vi "loop_transistor.vi"() -> ()   [LabVIEW 2020]
uses:
  <vilib>/Analysis/baseanly.llb/Mean (DBL).vi
  <vilib>/Utility/file.llb/Write Delimited Spreadsheet (DBL).vi
  <vilib>/Analysis/NI_AALBase.lvlib
panel:
  out "Isc [mA]":dbl
  out "Voc [V]":dbl
  out "resistance_MPP [kohm]":dbl
  out "resistance [kohm]":dbl
  in  "Save MPP operation data?":bool=TRUE
  out "MPP operating data log path":string
  in  "MPP operating\nfile name":string="MPP_operating"
  out "MPP tracking data log path":string
  in  "Save MPP tracking data?":bool=TRUE
  in  "MPP tracking\nfile name":string="MPP_tracking"
  in  "# points \nMPP operation":i32=6
  out "# iterations \nMPP operation (2nd loop)":dbl
  out "# iterations \nMPP tracking (1st loop)":i32
  out "error out":errorcluster
  out "Vgs_MPP [V]":dbl
  out "V_MPP [V]":dbl
  out "I_MPP [mA]":dbl
  out "index max power":i32
  out "max power [mW]":dbl
  in  "STOP":bool
  out "power [mW]":dbl
  in  "Tab Control":T1(tab)
  out "IV-PV":cluster{dbl[], dbl[]}[](graph)
  out "Power":dbl[](graph)
  out "Resistance-Vgs":cluster{dbl[], dbl[]}(graph)
  out "I,V (Vgs)":cluster{dbl[], dbl[]}[](graph)
  out "IV-PV":cluster{dbl[], dbl[]}[](graph)
  out "Current-Voltage-Power operating":dbl[][](graph)
  out "voltage [V]":dbl format="%0.2f"
  out "current [mA]":dbl
  in  "# points\nMPP tracking":i32=3
  out "Vgs [V]":dbl
  in  "Vgs stop":dbl=4.0 format="%#_13g"
  in  "Vgs step":dbl=0.05 format="%#_13g"
  in  "Vgs start":dbl=3.0 format="%#_13g"
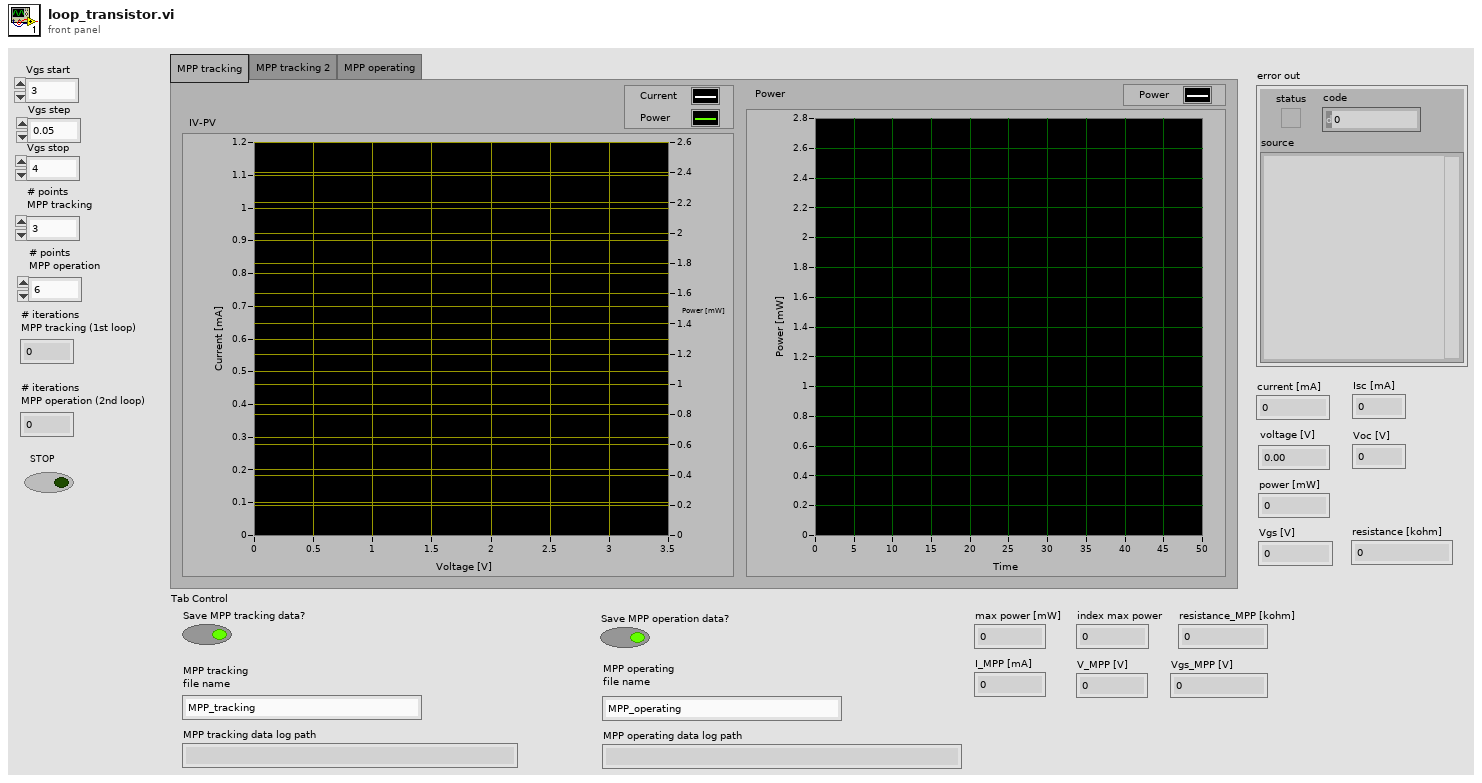
[diagram p1: front panel]
types:
  T1 = enum32{"MPP tracking", "MPP tracking 2", "MPP operating"}
  T2 = enum16{"open", "replace", "create", "open or create", "replace or create", "replace or create with confirmation"}
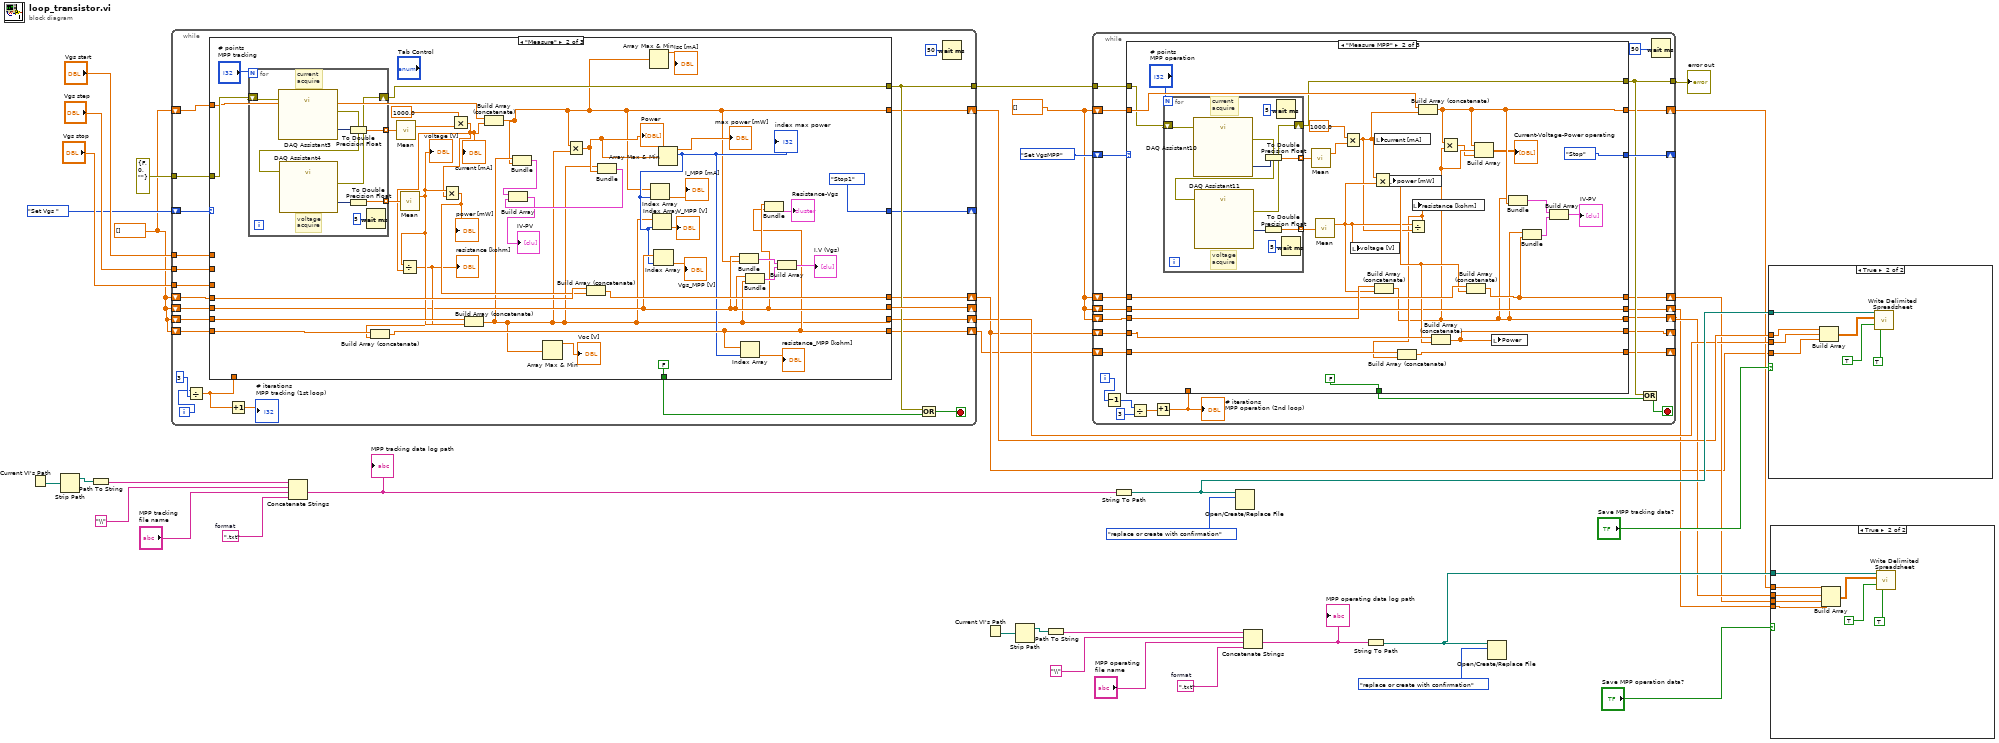
[diagram p0: block diagram]
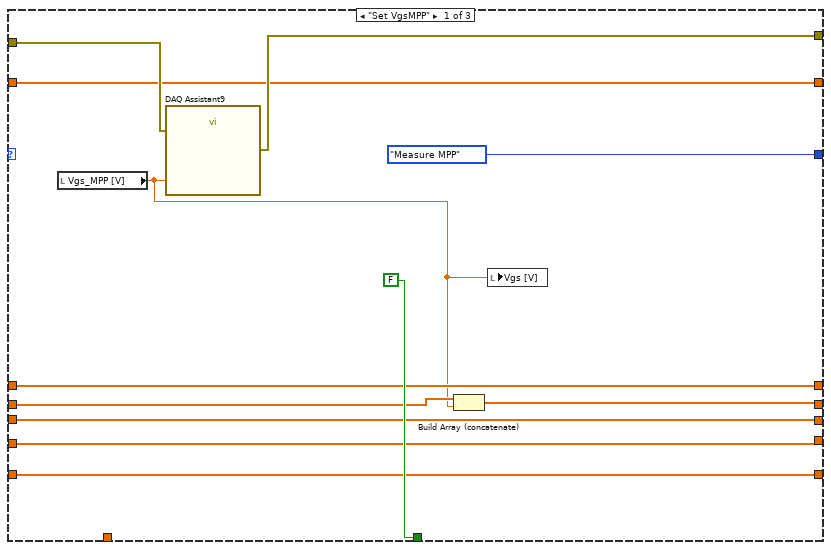
[diagram p4: hidden frame]
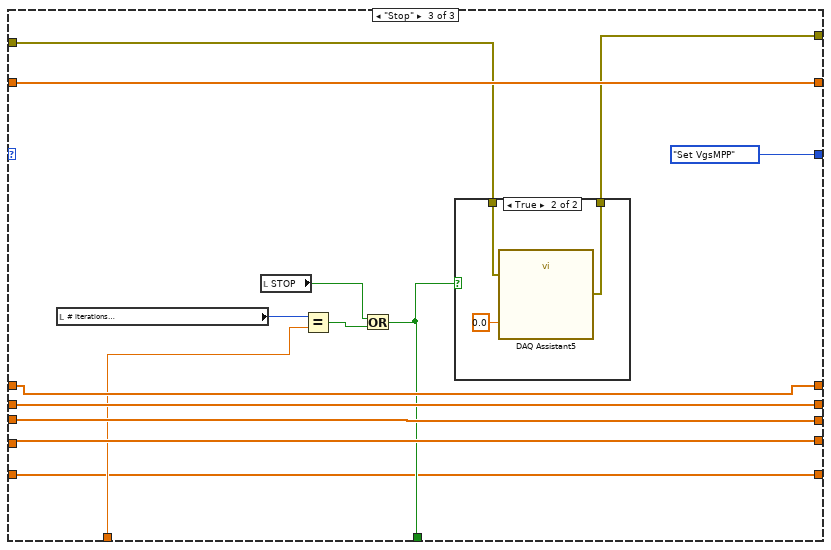
[diagram p5: hidden frame]
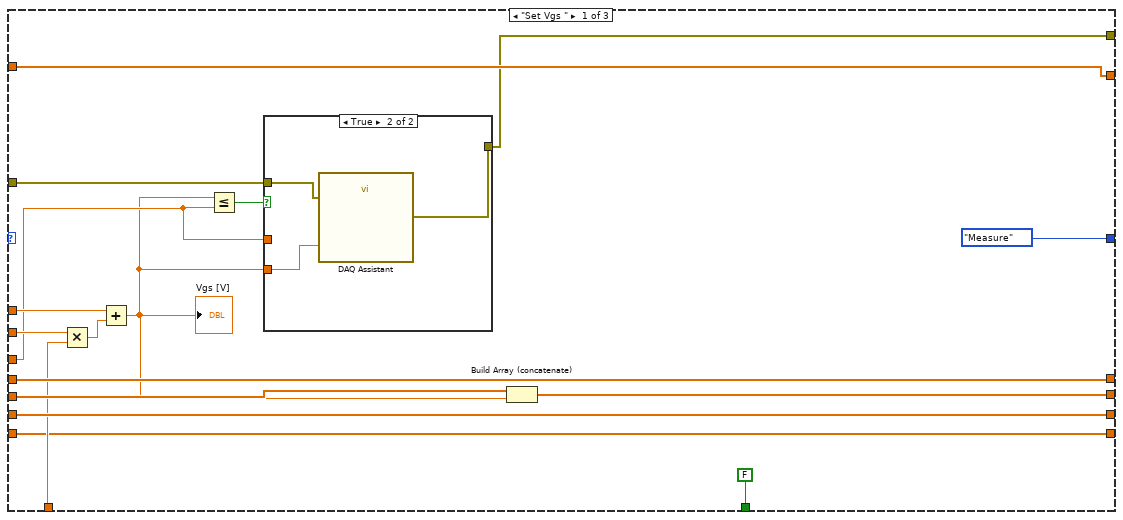
[diagram p7: hidden frame]
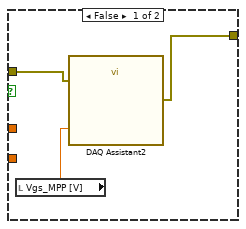
[diagram p8: hidden frame]
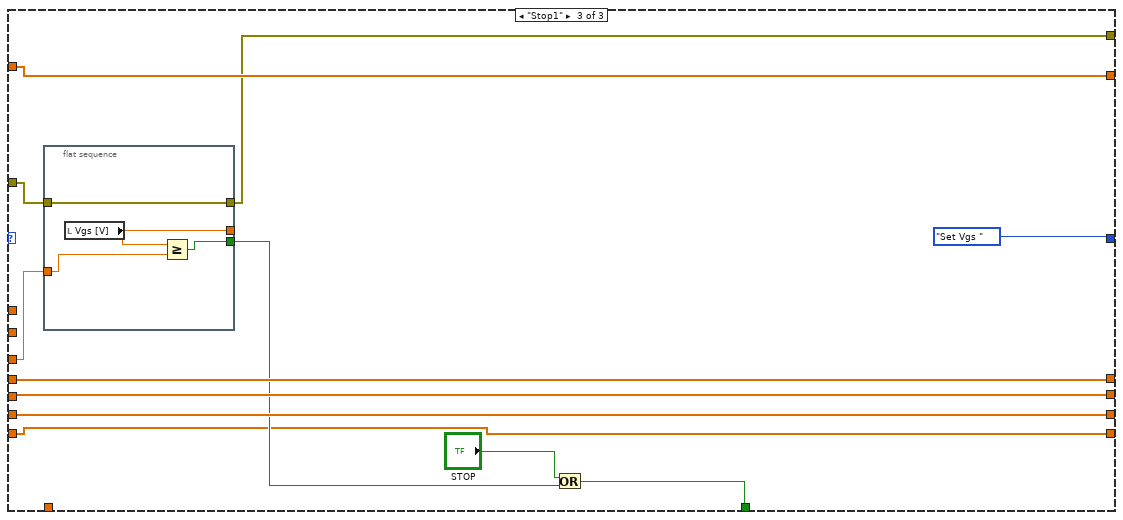
[diagram p9: hidden frame]
diagram:
  w14 = ".txt"  # format
  w26 = ".txt"  # format
  w32 = dbl[] []
  w2 = dbl[] []
  n1 = Current VI's Path() -> (path=w18:path)
  n2 = Strip Path(path=w18) -> (stripped path=w19:path)  [unwired: 1 out]
  n3 = Path To String(path=w19) -> (string=w29:string)
  n4 = while {
    tunnel: "Vgs start" -> [w62]
    tunnel: "Vgs step" -> [w61]
    tunnel: "Vgs stop" -> [w60]
    tunnel: errorcluster {"status"=FALSE, "code"=0, "source"=""} ("error in") -> [w59]
    tunnel: [w55] -> w31
    shift-right: [w57] -> _
    shift-left: w2 -> [w58]
    shift-right: [w45] -> _
    shift-left: enum16{"Set Vgs ", "Measure", "Stop1"}."Set Vgs " -> [w52]
    shift-right: [w50] -> w21
    shift-left: w2 -> [w51]
    shift-right: [w48] -> w20
    shift-left: w2 -> [w49]
    shift-right: [w46] -> w3
    shift-left: w2 -> [w47]
    shift-right: [w39] -> w1
    shift-left: w2 -> [w40]
    i -> [w43]
    stop <- w56 stop-if-true
    n5 = Divide(x=w43, y=3) -> (x/y=w41:dbl)
    n6 = case shown="\"Measure\"" w52 {
      tunnel: [enum16{"Set Vgs ", "Measure", "Stop1"}."Measure" enum16{"Set Vgs ", "Measure", "Stop1"}."Stop1" enum16{"Set Vgs ", "Measure", "Stop1"}."Set Vgs "] -> w45
      tunnel: w62 -> [w77 _ _]
      tunnel: w61 -> [w79 _ _]
      tunnel: w60 -> [w67 _ w141]
      tunnel: w41 -> [w66 _ _]
      tunnel: w59 -> [w75 w121 w140]
      tunnel: [w64 w122 w133] -> w55
      tunnel: w58 -> [w74 w94 w138]
      tunnel: [w73 w94 w138] -> w57
      tunnel: [FALSE FALSE w134] -> w54
      tunnel: w51 -> [w70 w116 w143]
      tunnel: [w70 w87 w143] -> w50
      tunnel: w49 -> [w71 w115 w137]
      tunnel: [w71 w89 w137] -> w48
      tunnel: w47 -> [w69 w110 w139]
      tunnel: [w69 w108 w139] -> w46
      tunnel: w40 -> [w63 w96 w132]
      tunnel: [w63 w92 w132] -> w39
      frame "Set Vgs " {
        n7 = Multiply(x=w79, y=w66) -> (x*y=w78:dbl)
        n8 = Add(x=w77, y=w78) -> (x+y=w65:dbl)
        "Vgs [V]" <- w65
        n9 = Less Or Equal?(x=w65, y=w67) -> (x <= y?=w76:bool)
        n10 = case shown="True" w76 {
          tunnel: w65 -> [_ w85]
          tunnel: w75 -> [w82 w84]
          tunnel: w67 -> [_ _]
          tunnel: [w81 w83] -> w64
          frame False {
            n11 = local read "Vgs_MPP [V]"() -> (w80:dbl)
            n12 = call "DAQ Assistant2"("data"=w80, "error in"=w82) -> ("error out"=w81:errorcluster)  [unwired: 16 in, 1 out]
          }
          frame True {
            n13 = call "DAQ Assistant"("data"=w85, "error in"=w84) -> ("error out"=w83:errorcluster)  [unwired: 16 in, 1 out]
          }
        }
        n14 = Build Array (concatenate)(w74, w65) -> (w73:dbl[])
      }
      frame "Measure" {
        n15 = for {
          N: "# points\nMPP tracking" -> [_]
          shift-right: [w130] -> w122
          shift-left: w121 -> [w126]
          tunnel: [w125] -> w120 mode=indexing
          tunnel: [w124] -> w117 mode=indexing
          # "voltage\nacquire"
          # "current \nacquire"
          n16 = call "DAQ Assistant3"("error in"=w126) -> ("data"=w128:dynamicdata, "error out"=w131:errorcluster)  [unwired: 16 in, 1 out]
          n17 = call "DAQ Assistant4"("error in"=w131) -> ("data"=w127:dynamicdata, "error out"=w130:errorcluster)  [unwired: 16 in, 1 out]
          n18 = To Double Precision Float(number=w128) -> (double precision float=w125:dbl)
          n19 = To Double Precision Float(number=w127) -> (double precision float=w124:dbl)
          n20 = Wait (ms)(milliseconds to wait=u32 5) -> ()  [unwired: 1 out]
        }
        n21 = call-poly <vilib>:"Mean.vi"("X"=w120) -> ("mean"=w119:dbl)  [unwired: 1 out]
        n22 = call-poly <vilib>:"Mean.vi"("X"=w117) -> ("mean"=w98:dbl)  [unwired: 1 out]
        "voltage [V]" <- w98
        n23 = Multiply(x=1000.0, y=w119) -> (x*y=w97:dbl)
        "current [mA]" <- w97
        n24 = Divide(x=w98, y=w97) -> (x/y=w95:dbl)
        "resistance [kohm]" <- w95
        n25 = Build Array (concatenate)(w96, w95) -> (w92:dbl[])
        n26 = Multiply(x=w98, y=w97) -> (x*y=w109:dbl)
        "power [mW]" <- w109
        n27 = Build Array (concatenate)(w115, w98) -> (w89:dbl[])
        n28 = Build Array (concatenate)(w116, w97) -> (w87:dbl[])
        n29 = Bundle(w89, w87) -> (w114:cluster{dbl[], dbl[]})  [unwired: 1 in]
        n30 = Array Max & Min(array=w89) -> (max value=→"Voc [V]":dbl)  [unwired: 3 out]
        n31 = Multiply(x=w87, y=w89) -> (x*y=w102:dbl[])
        "Power" <- w102
        n32 = Build Array (concatenate)(w110, w109) -> (w108:dbl[])
        n33 = Bundle(w89, w102) -> (w113:cluster{dbl[], dbl[]})  [unwired: 1 in]
        n34 = Build Array(w114, w113) -> (→"IV-PV":cluster{dbl[], dbl[]}[])
        n35 = Array Max & Min(array=w87) -> (max value=→"Isc [mA]":dbl)  [unwired: 3 out]
        n36 = Array Max & Min(array=w102) -> (max value=→"max power [mW]":dbl, max index (indices)=w91:i32)  [unwired: 2 out]
        "index max power" <- w91
        n37 = Index Array(array=w87, index=w91) -> (element=→"I_MPP [mA]":dbl)
        n38 = Index Array(array=w89, index=w91) -> (element=→"V_MPP [V]":dbl)
        n39 = Index Array(array=w94, index=w91) -> (element=→"Vgs_MPP [V]":dbl)
        n40 = Bundle(w94, w87) -> (w101:cluster{dbl[], dbl[]})  [unwired: 1 in]
        n41 = Index Array(array=w92, index=w91) -> (element=→"resistance_MPP [kohm]":dbl)
        n42 = Bundle(w94, w89) -> (w100:cluster{dbl[], dbl[]})  [unwired: 1 in]
        n43 = Bundle(w94, w92) -> (→"Resistance-Vgs":cluster{dbl[], dbl[]})  [unwired: 1 in]
        n44 = Build Array(w101, w100) -> (→"I,V (Vgs)":cluster{dbl[], dbl[]}[])
      }
      frame "Stop1" {
        n45 = flat-sequence {
          tunnel: w141 -> [w147]
          tunnel: [w146] -> w135
          tunnel: [w145] -> _
          tunnel: w140 -> [w144]
          tunnel: [w144] -> w133
          frame #0 {
            n46 = local read "Vgs [V]"() -> (w145:dbl)
            n47 = Greater Or Equal?(x=w145, y=w147) -> (x >= y?=w146:bool)
          }
        }
        n48 = Or(x="STOP", y=w135) -> (x .or. y?=w134:bool)
      }
    }
    n49 = Increment(x=w41) -> (x+1=→"# iterations \nMPP tracking (1st loop)":dbl)
    n50 = Or(x=w55, y=w54) -> (x .or. y?=w56:bool)
    n51 = Wait (ms)(milliseconds to wait=u32 50) -> ()  [unwired: 1 out]
  }
  n52 = Concatenate Strings(w29, "\\" ("string"), "MPP tracking\nfile name", w26) -> (w25:string)
  "MPP tracking data log path" <- w25
  n53 = Current VI's Path() -> (path=w12:path)
  n54 = Strip Path(path=w12) -> (stripped path=w13:path)  [unwired: 1 out]
  n55 = Path To String(path=w13) -> (string=w17:string)
  n56 = while {
    shift-right: [w170] -> _
    shift-left: enum16{"Set VgsMPP", "Measure MPP", "Stop"}."Set VgsMPP" -> [w171]
    tunnel: [w167] -> w30
    tunnel: w31 -> [w166]
    shift-right: [w164] -> w5
    shift-left: w32 -> [w165]
    shift-right: [w163] -> w6
    shift-left: w32 -> [w162]
    shift-right: [w160] -> w7
    shift-left: w32 -> [w161]
    shift-right: [w158] -> w4
    shift-left: w32 -> [w159]
    shift-right: [w152] -> _
    shift-left: w3 -> [w153]
    shift-right: [w148] -> _
    shift-left: w1 -> [w149]
    i -> [w154]
    stop <- w168 stop-if-true
    n57 = Decrement(x=w154) -> (x-1=w155:i32)
    n58 = Divide(x=w155, y=3) -> (x/y=w156:dbl)
    n59 = Increment(x=w156) -> (x+1=w151:dbl)
    "# iterations \nMPP operation (2nd loop)" <- w151
    n60 = case shown="\"Measure MPP\"" w171 {
      tunnel: [enum16{"Set VgsMPP", "Measure MPP", "Stop"}."Measure MPP" enum16{"Set VgsMPP", "Measure MPP", "Stop"}."Stop" enum16{"Set VgsMPP", "Measure MPP", "Stop"}."Set VgsMPP"] -> w170
      tunnel: [w182 w204 w229] -> w167
      tunnel: [FALSE FALSE w223] -> w150
      tunnel: w166 -> [w180 w202 w230]
      tunnel: [w179 w197 w233] -> w164
      tunnel: w165 -> [w179 w203 w233]
      tunnel: [w178 w186 w232] -> w163
      tunnel: w162 -> [w178 w205 w232]
      tunnel: [w177 w187 w234] -> w160
      tunnel: w161 -> [w177 w206 w234]
      tunnel: w159 -> [w176 w189 w231]
      tunnel: [w175 w189 w231] -> w158
      tunnel: w153 -> [w173 w196 w228]
      tunnel: [w173 w194 w228] -> w152
      tunnel: w151 -> [_ _ w226]
      tunnel: w149 -> [w172 w191 w222]
      tunnel: [w172 w188 w222] -> w148
      frame "Set VgsMPP" {
        n61 = local read "Vgs_MPP [V]"() -> (w174:dbl)
        n62 = call "DAQ Assistant9"("data"=w174, "error in"=w180) -> ("error out"=w182:errorcluster)  [unwired: 16 in, 1 out]
        n63 = Build Array (concatenate)(w176, w174) -> (w175:dbl[])
        n64 = local write "Vgs [V]"(w174) -> ()
      }
      frame "Measure MPP" {
        n65 = for {
          N: "# points \nMPP operation" -> [_]
          shift-right: [w220] -> w204
          shift-left: w202 -> [w216]
          tunnel: [w215] -> w207 mode=indexing
          tunnel: [w214] -> w208 mode=indexing
          # "voltage\nacquire"
          # "current \nacquire"
          n66 = call "DAQ Assistant10"("error in"=w216) -> ("data"=w218:dynamicdata, "error out"=w221:errorcluster)  [unwired: 16 in, 1 out]
          n67 = call "DAQ Assistant11"("error in"=w221) -> ("data"=w217:dynamicdata, "error out"=w220:errorcluster)  [unwired: 16 in, 1 out]
          n68 = To Double Precision Float(number=w218) -> (double precision float=w215:dbl)
          n69 = To Double Precision Float(number=w217) -> (double precision float=w214:dbl)
          n70 = Wait (ms)(milliseconds to wait=u32 5) -> ()  [unwired: 1 out]
          n71 = Wait (ms)(milliseconds to wait=u32 5) -> ()  [unwired: 1 out]
        }
        n72 = call-poly <vilib>:"Mean.vi"("X"=w207) -> ("mean"=w209:dbl)  [unwired: 1 out]
        n73 = call-poly <vilib>:"Mean.vi"("X"=w208) -> ("mean"=w193:dbl)  [unwired: 1 out]
        n74 = Multiply(x=1000.0, y=w209) -> (x*y=w192:dbl)
        n75 = local write "voltage [V]"(w193) -> ()
        n76 = Multiply(x=w192, y=w193) -> (x*y=w195:dbl)
        n77 = local write "current [mA]"(w192) -> ()
        n78 = Build Array (concatenate)(w205, w193) -> (w186:dbl[])
        n79 = local write "power [mW]"(w195) -> ()
        n80 = Divide(x=w193, y=w192) -> (x/y=w190:dbl)
        n81 = Build Array (concatenate)(w191, w190) -> (w188:dbl[])
        n82 = local write "resistance [kohm]"(w190) -> ()
        n83 = Build Array (concatenate)(w206, w192) -> (w187:dbl[])
        n84 = Build Array (concatenate)(w196, w195) -> (w194:dbl[])
        n85 = Multiply(x=w187, y=w186) -> (x*y=w185:dbl[])
        n86 = Build Array (concatenate)(w203, w195) -> (w197:dbl[])
        n87 = Build Array(w187, w186, w185) -> (→"Current-Voltage-Power operating":dbl[][])
        n88 = local write "Power"(w194) -> ()
        n89 = Bundle(w186, w187) -> (w200:cluster{dbl[], dbl[]})  [unwired: 1 in]
        n90 = Bundle(w186, w197) -> (w199:cluster{dbl[], dbl[]})  [unwired: 1 in]
        n91 = Build Array(w200, w199) -> (→"IV-PV":cluster{dbl[], dbl[]}[])
      }
      frame "Stop" {
        n92 = local read "# iterations \nMPP tracking (1st loop)"() -> (w227:i32)
        n93 = local read "STOP"() -> (w225:bool)
        n94 = Equal?(x=w227, y=w226) -> (x = y?=w224:bool)
        n95 = Or(x=w225, y=w224) -> (x .or. y?=w223:bool)
        n96 = case shown="True" w223 {
          tunnel: w230 -> [w236 w239]
          tunnel: [w236 w238] -> w229
          frame False {
          }
          frame True {
            n97 = call "DAQ Assistant5"("data"=0.0, "error in"=w239) -> ("error out"=w238:errorcluster)  [unwired: 16 in, 1 out]
          }
        }
      }
    }
    n98 = Or(x=w167, y=w150) -> (x .or. y?=w168:bool)
    n99 = Wait (ms)(milliseconds to wait=u32 50) -> ()  [unwired: 1 out]
  }
  "error out" <- w30
  n100 = String To Path(string=w25) -> (path=w22:path)
  n101 = Open/Create/Replace File(file path (use dialog)=w22, operation (0:open)=T2."replace or create with confirmation") -> ()  [unwired: 4 in, 3 out]
  n102 = Concatenate Strings(w17, "\\" ("string"), "MPP operating\nfile name", w14) -> (w10:string)
  "MPP operating data log path" <- w10
  n103 = String To Path(string=w10) -> (path=w8:path)
  n104 = Open/Create/Replace File(file path (use dialog)=w8, operation (0:open)=T2."replace or create with confirmation") -> ()  [unwired: 4 in, 3 out]
  n105 = case shown="True" "Save MPP tracking data?" {
    tunnel: w22 -> [_ w246]
    tunnel: w21 -> [_ w245]
    tunnel: w20 -> [_ w244]
    tunnel: w3 -> [_ w243]
    frame False {
    }
    frame True {
      n106 = Build Array(w245, w244, w243) -> (w242:dbl[][])
      n107 = call-poly <vilib>:"Write Delimited Spreadsheet.vi"("file path (dialog if empty)"=w246, "2D data"=w242, "append to file? (new file:F)"=TRUE, "transpose? (no:F)"=TRUE) -> ()  [unwired: 10 in, 2 out]
    }
  }
  n108 = case shown="True" "Save MPP operation data?" {
    tunnel: w8 -> [_ w252]
    tunnel: w7 -> [_ w251]
    tunnel: w6 -> [_ w250]
    tunnel: w5 -> [_ w249]
    tunnel: w4 -> [_ w247]
    frame False {
    }
    frame True {
      n109 = Build Array(w251, w250, w249, w247) -> (w248:dbl[][])
      n110 = call-poly <vilib>:"Write Delimited Spreadsheet.vi"("file path (dialog if empty)"=w252, "2D data"=w248, "append to file? (new file:F)"=TRUE, "transpose? (no:F)"=TRUE) -> ()  [unwired: 10 in, 2 out]
    }
  }
